vi "Battery Logging.vi"() -> ()   [LabVIEW 2015]
uses:
  <vilib>/DAQmx/read.llb/DAQmx Read.vi
  <vilib>/DAQmx/read.llb/DAQmx Read (Analog 1D DBL 1Chan NSamp).vi
  <vilib>/DAQmx/miscellaneous.llb/DAQmx Fill In Error Info.vi
panel:
  out "data":dbl[](graph)
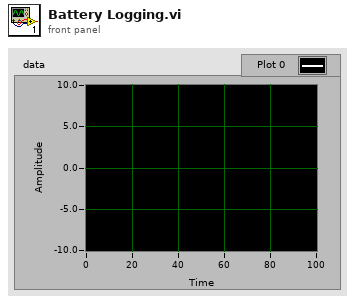
[diagram p1: front panel]
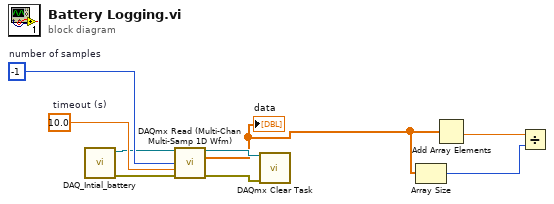
[diagram p0: block diagram]
diagram:
  w8 = 10.0  # timeout (s)
  w9 = -1  # number of samples
  n1 = call "DAQ_Intial_battery.vi"() -> ("error out"=w4:errorcluster, "task out"=w5:refnum<k21>)  [unwired: 10 in]
  n2 = call-poly "DAQmx Read (Multi-Chan Multi-Samp 1D Wfm).vi"("task/channels in"=w5, "number of samples per channel"=w9, "timeout"=w8, "error in"=w4) -> ("task out"=w6:refnum<k21>, "data"=w2:dbl[], "error out"=w7:errorcluster)  [unwired: 9 in]
  "data" <- w2
  n3 = call <vilib>:"DAQmx Clear Task.vi"("task in"=w6, "error in"=w7) -> ()  [unwired: 13 in, 1 out]
  n4 = Array Size(array=w2) -> (size(s)=w1:i32)
  n5 = Add Array Elements(numeric array=w2) -> (sum=w3:dbl)
  n6 = Divide(x=w3, y=w1) -> ()  [unwired: 1 out]
